vi "V to Temperature converter.vi"(1 "Waveform":dbl) -> (0 "Numeric":dbl)   [LabVIEW 2022 SP3]
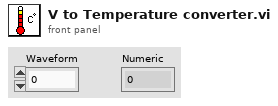
[diagram p1: front panel]
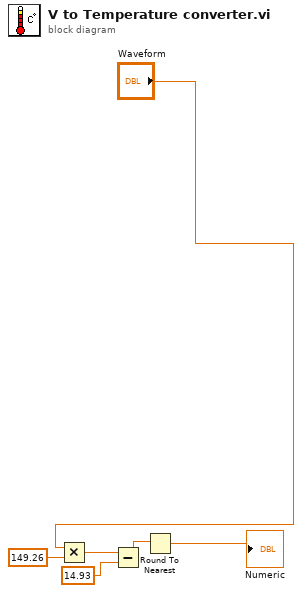
[diagram p0: block diagram]
diagram:
  n1 = Multiply(x="Waveform", y=149.26) -> (x*y=w3:dbl)
  n2 = Subtract(x=w3, y=14.93) -> (x-y=w5:dbl)
  n3 = Round To Nearest(number=w5) -> (nearest integer value=→"Numeric":dbl)
